vi "Register Data Logging Events.vi"(8 "error in (no error)":errorcluster, 11 "Data Logging Manager Ref in":T4) -> (0 "error out":errorcluster, 3 "Data Logging Manager Ref out":T4, 4 "Log Event Registration Refnum":T1, 5 "Registered Data Logging Event Refnum":T2)   [LabVIEW 2020, in "NI_VS Data Logging API.lvlib"]
doc: "Registers for data logging events from the VeriStand Gateway. This VI returns a registered user event reference and information about the event."
uses:
  <vilib>/NI VeriStand/Execution/DataLogging/NI_VS Data Logging API.lvlib
  <vilib>/NI VeriStand/Execution/DataLogging/IDataLogging Ref.ctl
  NationalInstruments.VeriStand.ClientAPI
  <vilib>/NI VeriStand/Execution/DataLogging/Registered Data Logging Event Refnum.ctl
  <vilib>/NI VeriStand/Execution/DataLogging/Data Logging User Event Refs.ctl
  <vilib>/NI VeriStand/Execution/DataLogging/Data Logging Session Error Event Data.ctl
  <vilib>/NI VeriStand/Execution/DataLogging/Data Logging Session Start Event Data.ctl
  <vilib>/NI VeriStand/Execution/DataLogging/Data Logging Session State Change Event Data.ctl
  <vilib>/NI VeriStand/Execution/DataLogging/Data Logging Session State.ctl
  <vilib>/NI VeriStand/Execution/DataLogging/Data Logging Session Stop Event Data.ctl
  <vilib>/NI VeriStand/Execution/DataLogging/Log File Closed Event Data.ctl
  <vilib>/NI VeriStand/Execution/DataLogging/Log File Opened Event Data.ctl
  <vilib>/NI VeriStand/Execution/DataLogging/New Log Files Complete Event Data.ctl
  <vilib>/NI VeriStand/Execution/DataLogging/Data Logging Event Registration Refnum.ctl
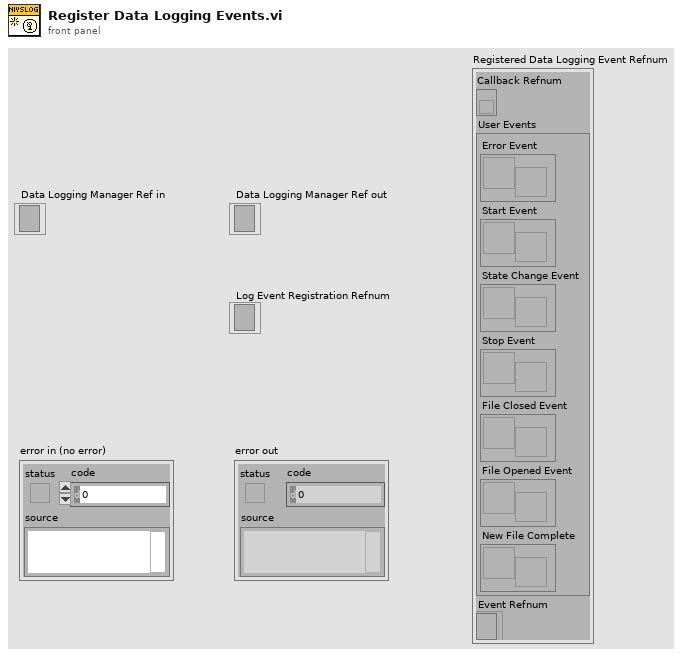
[diagram p1: front panel]
types:
  T1 = typedef "NI_VS Data Logging API.lvlib/Data Logging Event Registration Refnum.ctl" = refnum<event-registration>
  T2 = typedef "NI_VS Data Logging API.lvlib/Registered Data Logging Event Refnum.ctl" = cluster{"Callback Refnum":refnum<k27>, "User Events":T3, "Event Refnum":T1}
  T3 = typedef "NI_VS Data Logging API.lvlib/Data Logging User Event Refs.ctl" = cluster{"Error Event":refnum<user-event>, "Start Event":refnum<user-event>, "State Change Event":refnum<user-event>, "Stop Event":refnum<user-event>, "File Closed Event":refnum<user-event>, "File Opened Event":refnum<user-event>, "New File Complete":refnum<user-event>}
  T4 = typedef "NI_VS Data Logging API.lvlib/IDataLogging Ref.ctl" = refnum<k24>
  T5 = typedef "NI_VS Data Logging API.lvlib/New Log Files Complete Event Data.ctl" = cluster{"Log File Paths":path[], "Log File Source":string, "Target":string}
  T6 = typedef "NI_VS Data Logging API.lvlib/Log File Opened Event Data.ctl" = cluster{"Session Name":string, "Log File Path":path}
  T7 = typedef "NI_VS Data Logging API.lvlib/Log File Closed Event Data.ctl" = cluster{"Session Name":string, "Log File Path":path}
  T8 = typedef "NI_VS Data Logging API.lvlib/Data Logging Session Stop Event Data.ctl" = cluster{"Session Name":string, "Log File Paths":path[]}
  T9 = typedef "NI_VS Data Logging API.lvlib/Data Logging Session State Change Event Data.ctl" = cluster{"Session Name":string, "Session State":T10}
  T10 = typedef "NI_VS Data Logging API.lvlib/Data Logging Session State.ctl" = enum16{"Waiting on Trigger", "Triggered", "Post-Trigger", "Complete", "Idle", "Error"}
  T11 = typedef "NI_VS Data Logging API.lvlib/Data Logging Session Start Event Data.ctl" = cluster{"Session Name":string}
  T12 = typedef "NI_VS Data Logging API.lvlib/Data Logging Session Error Event Data.ctl" = cluster{"Session Name":string, "Error":errorcluster}
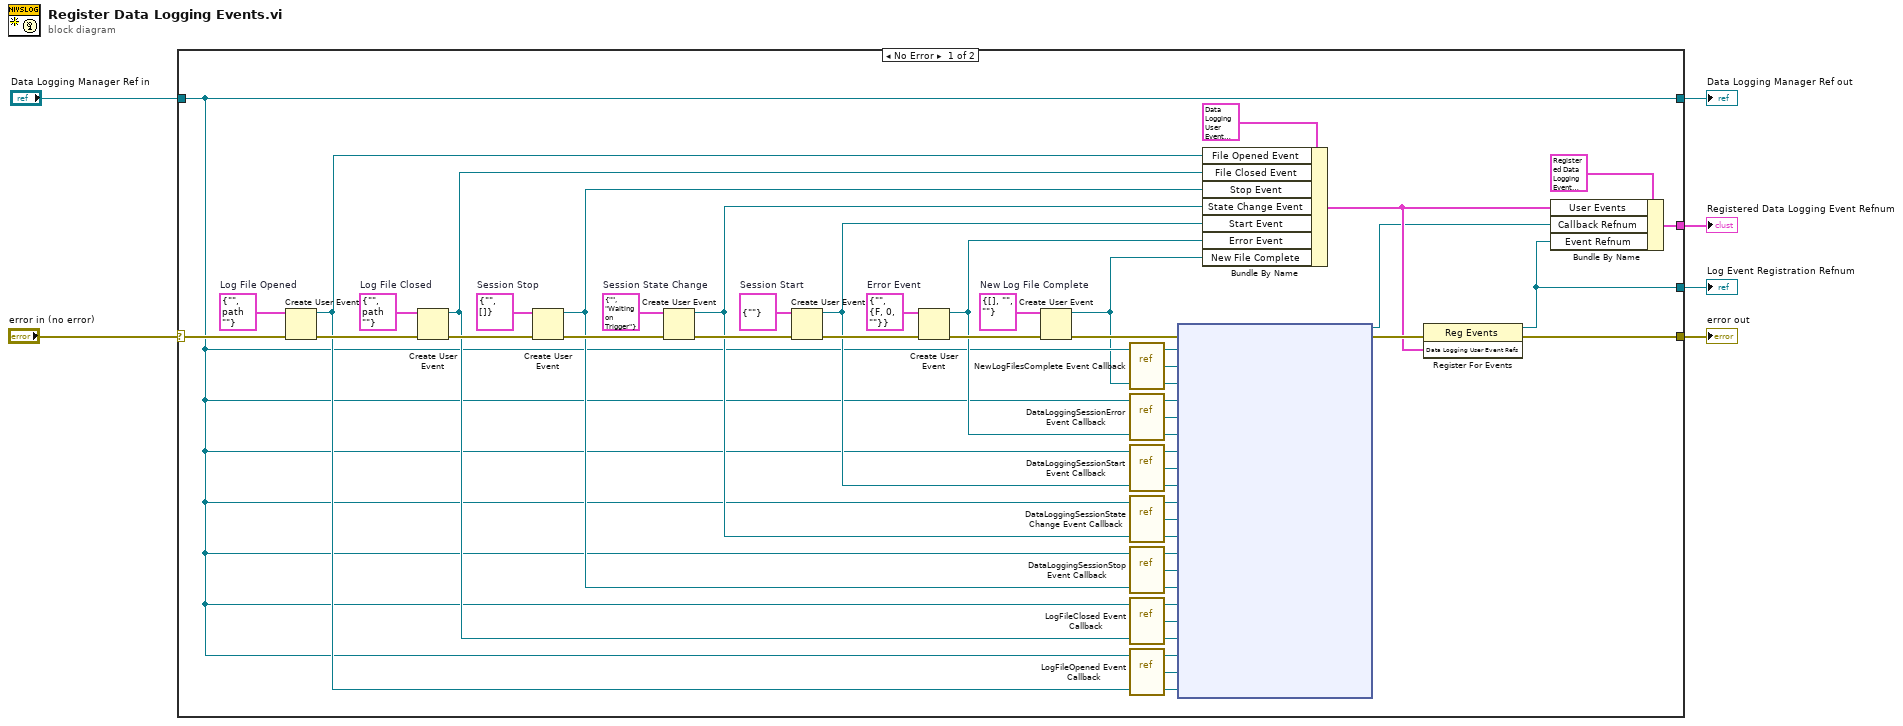
[diagram p0: block diagram]
diagram:
  n1 = case shown="No Error" "error in (no error)" {
    selector: "error in (no error)" -> [w32 w45]
    tunnel: [w14 w45] -> w6
    tunnel: "Data Logging Manager Ref in" -> [w10 w46]
    tunnel: [w10 w46] -> w3
    tunnel: [w13 _] -> w2
    tunnel: [w12 _] -> w1
    frame No Error {
      w11 = T5 {"Log File Paths"=[], "Log File Source"="", "Target"=""}  # New Log File Complete
      w33 = T6 {"Session Name"="", "Log File Path"=path ""}  # Log File Opened
      w35 = T7 {"Session Name"="", "Log File Path"=path ""}  # Log File Closed
      w37 = T8 {"Session Name"="", "Log File Paths"=[]}  # Session Stop
      w39 = T9 {"Session Name"="", "Session State"=enum."Waiting on Trigger"}  # Session State Change
      w41 = T11 {"Session Name"=""}  # Session Start
      w42 = T12 {"Session Name"="", "Error"={"status"=FALSE, "code"=0, "source"=""}}  # Error Event
      n2 = Create User Event(user event datatype=w33, error in=w32) -> (user event=w26:refnum<user-event>, error out=w34:errorcluster)
      n3 = Create User Event(user event datatype=w35, error in=w34) -> (user event=w27:refnum<user-event>, error out=w36:errorcluster)
      n4 = Create User Event(user event datatype=w37, error in=w36) -> (user event=w28:refnum<user-event>, error out=w38:errorcluster)
      n5 = Create User Event(user event datatype=w39, error in=w38) -> (user event=w29:refnum<user-event>, error out=w40:errorcluster)
      n6 = Create User Event(user event datatype=w41, error in=w40) -> (user event=w30:refnum<user-event>, error out=w43:errorcluster)
      n7 = Create User Event(user event datatype=w42, error in=w43) -> (user event=w31:refnum<user-event>, error out=w44:errorcluster)
      n8 = Create User Event(user event datatype=w11, error in=w44) -> (user event=w8:refnum<user-event>, error out=w9:errorcluster)
      n9 = vi-ref <vilib>:"NewLogFilesComplete Event Callback.vi"() -> ("vi reference"=w7:refnum<vi>)
      n10 = vi-ref <vilib>:"DataLoggingSessionError Event Callback.vi"() -> ("vi reference"=w25:refnum<vi>)
      n11 = vi-ref <vilib>:"DataLoggingSessionStart Event Callback.vi"() -> ("vi reference"=w24:refnum<vi>)
      n12 = vi-ref <vilib>:"DataLoggingSessionStateChange Event Callback.vi"() -> ("vi reference"=w23:refnum<vi>)
      n13 = vi-ref <vilib>:"DataLoggingSessionStop Event Callback.vi"() -> ("vi reference"=w22:refnum<vi>)
      n14 = vi-ref <vilib>:"LogFileClosed Event Callback.vi"() -> ("vi reference"=w21:refnum<vi>)
      n15 = vi-ref <vilib>:"LogFileOpened Event Callback.vi"() -> ("vi reference"=w20:refnum<vi>)
      n16 = node(w9, w10, w7, w8, w10, w25, w31, w10, w24, w30, w10, w23, w29, w10, w22, w28, w10, w21, w27, w10, w20, w26) -> (w15:refnum<k27>, w18:errorcluster)  [unwired: 1 in]
      n17 = Bundle By Name(cluster=T3 {"Error Event"=refnum, "Start Event"=refnum, "State Change Event"=refnum, "Stop Event"=refnum, "File Closed Event"=refnum, "File Opened Event"=refnum, "New File Complete"=refnum} ("Data Logging User Event Refs"), "File Opened Event"=w26, "File Closed Event"=w27, "Stop Event"=w28, "State Change Event"=w29, "Start Event"=w30, "Error Event"=w31, "New File Complete"=w8) -> (w16:T3)
      n18 = register-events(error in=w18, w16) -> (reference out=w12:refnum<event-registration>, error out=w14:errorcluster)  [unwired: 1 in]
      n19 = Bundle By Name(cluster=T2 {"Callback Refnum"=refnum, "User Events"={"Error Event"=refnum, "Start Event"=refnum, "State Change Event"=refnum, "Stop Event"=refnum, "File Closed Event"=refnum, "File Opened Event"=refnum, "New File Complete"=refnum}, "Event Refnum"=refnum} ("Registered Data Logging Event Refnum"), "User Events"=w16, "Callback Refnum"=w15, "Event Refnum"=w12) -> (w13:T2)
    }
    frame Error {
    }
  }
  "Data Logging Manager Ref out" <- w3
  "error out" <- w6
  "Registered Data Logging Event Refnum" <- w2
  "Log Event Registration Refnum" <- w1
